vi "getCalRangeSelectionIndex.vi"(1 "calType":enum16{"INTERNAL_CAL", "FULL_CAL"}(ring)) -> (0 "range selection index":u32)   [LabVIEW 2024]
uses:
  Program Files (x86)/Luna Technologies/OVA 5000 v5.14.2/data/OVA32.dll
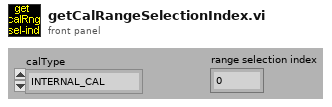
[diagram p1: front panel]
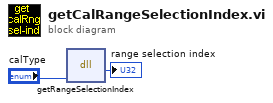
[diagram p0: block diagram]
diagram:
  n1 = dll-call lib="C:/Program Files (x86)/Luna Technologies/OVA 5000 v5.14.2/data/OVA32.dll" fn="getRangeSelectionIndex"("calType"="calType") -> (→"range selection index":u32)  [unwired: 4 in, 2 out]
